vi "Init.vi"(7 "BackPointer":refnum<data-value>, 8 "inOpen":bool, 9 "inClosed":i32, 10 "v":dbl=inf, 11 "g":dbl=inf) -> (3 "node ref out":refnum<data-value>)   [LabVIEW 2017, in "NI_Robotics_AbstractDstarNode.lvclass"]
uses:
  <vilib>/robotics/Navigation/shared/MapNode/AbstractDstarNode/NI_Robotics_AbstractDstarNode.lvclass
  <vilib>/robotics/Navigation/shared/MapNode/AbstractMapNode/NI_Robotics_AbstractMapNode.lvclass
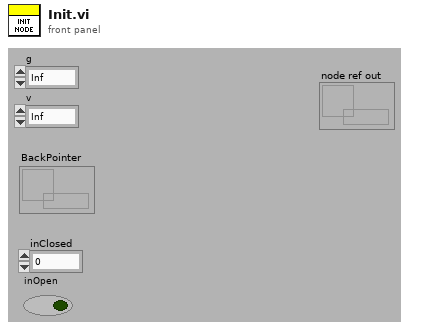
[diagram p1: front panel]
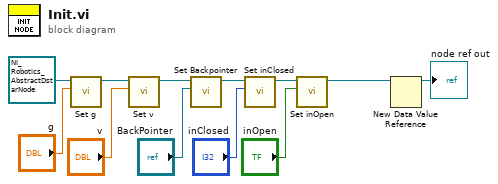
[diagram p0: block diagram]
diagram:
  n1 = call <vilib>:"Set g.vi"("g"="g", "AbstractDstarNode in"=refnum<class "NI_Robotics_AbstractDstarNode.lvclass"> refnum ("AbstractDstarNode.lvclass")) -> ("AbstractDstarNode out"=w11:refnum<class "NI_Robotics_AbstractDstarNode.lvclass">)  [unwired: 9 in]
  n2 = call <vilib>:"Set v.vi"("v"="v", "AbstractDstarNode in"=w11) -> ("AbstractDstarNode out"=w8:refnum<class "NI_Robotics_AbstractDstarNode.lvclass">)  [unwired: 9 in]
  n3 = call <vilib>:"Set Backpointer.vi"("BackPointer"="BackPointer", "AbstractDstarNode in"=w8) -> ("AbstractDstarNode out"=w7:refnum<class "NI_Robotics_AbstractDstarNode.lvclass">)  [unwired: 8 in, 1 out]
  n4 = call <vilib>:"Set inClosed.vi"("inClosed"="inClosed", "AbstractDstarNode in"=w7) -> ("AbstractDstarNode out"=w6:refnum<class "NI_Robotics_AbstractDstarNode.lvclass">)  [unwired: 8 in, 1 out]
  n5 = call <vilib>:"Set inOpen.vi"("inOpen"="inOpen", "AbstractDstarNode in"=w6) -> ("AbstractDstarNode out"=w2:refnum<class "NI_Robotics_AbstractDstarNode.lvclass">)  [unwired: 8 in, 1 out]
  n6 = New Data Value Reference(data value=w2) -> (data value reference=→"node ref out":refnum<data-value>)  [unwired: 1 in, 1 out]
